vi "set_folder_path.vi"(8 "error in (no error)":errorcluster, 10 "file path":path, 11 "Notebook.lvclass in":refnum<class "Notebook.lvclass">) -> (0 "error out":errorcluster, 3 "Notebook.lvclass out":refnum<class "Notebook.lvclass">)   [LabVIEW 2010, in "Notebook.lvclass"]
uses:
  Notebook.lvclass
  Notebook.lvclass/Notebook.ctl
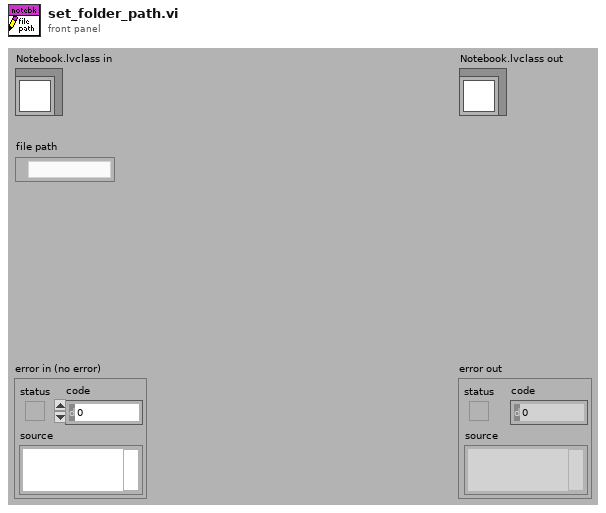
[diagram p1: front panel]
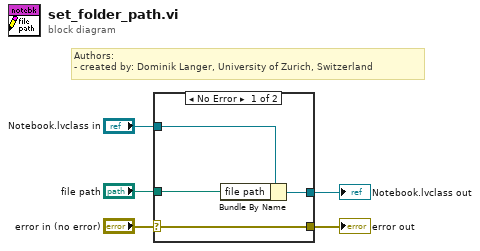
[diagram p0: block diagram]
diagram:
  # "Authors: \n- created by: Dominik Langer, University of Zurich, Switzerland"
  n1 = case shown="No Error" "error in (no error)" {
    selector: "error in (no error)" -> [w9 w10]
    tunnel: [w9 w10] -> w4
    tunnel: [w7 w11] -> w2
    tunnel: "Notebook.lvclass in" -> [w8 w11]
    tunnel: "file path" -> [w6 _]
    frame No Error {
      n2 = Bundle By Name(cluster=w8, "file path"=w6) -> (w7:refnum<class "Notebook.lvclass">)
    }
    frame Error {
    }
  }
  "error out" <- w4
  "Notebook.lvclass out" <- w2
